vi "D2SParser - Private - Function - Open File.vi"(8 "error in (no error)":errorcluster, 10 "Path":path, 11 "D2SParser in":refnum<class "D2SParser.lvclass">) -> (0 "error out":errorcluster, 3 "D2SParser out":refnum<class "D2SParser.lvclass">)   [LabVIEW 2015, in "D2SParser.lvclass"]
uses:
  D2SParser.lvclass
  D2SParser.lvclass/D2SParser.ctl
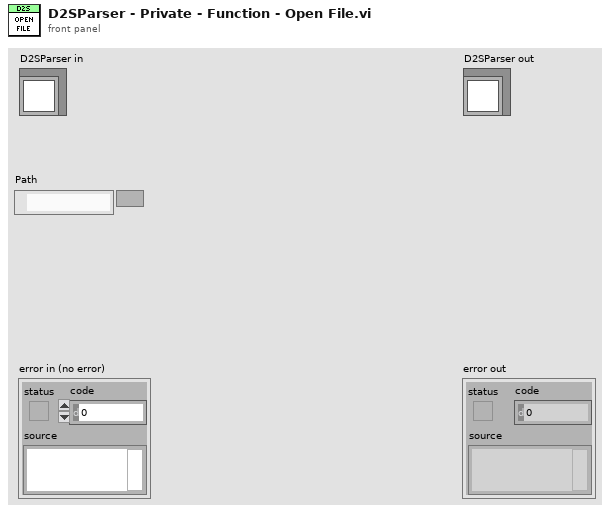
[diagram p1: front panel]
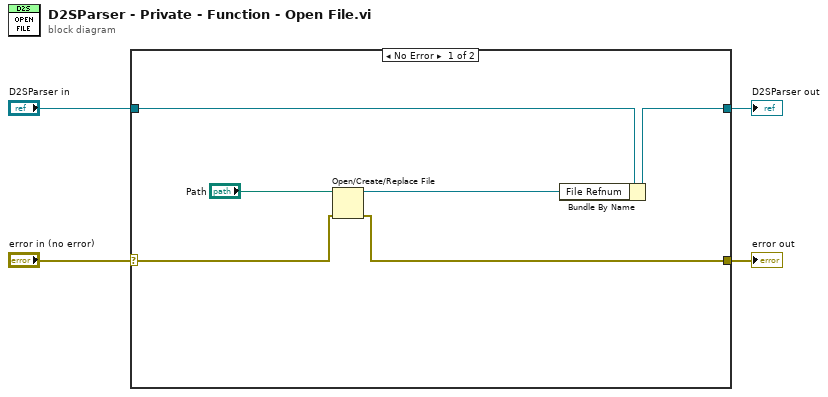
[diagram p0: block diagram]
diagram:
  n1 = case shown="No Error" "error in (no error)" {
    selector: "error in (no error)" -> [w8 w12]
    tunnel: [w7 w12] -> w3
    tunnel: [w6 w11] -> w1
    tunnel: "D2SParser in" -> [w10 w11]
    frame No Error {
      n2 = Open/Create/Replace File(file path (use dialog)="Path", error in=w8) -> (refnum out=w5:refnum<file>, error out=w7:errorcluster)  [unwired: 4 in, 1 out]
      n3 = Bundle By Name(cluster=w10, "File Refnum"=w5) -> (w6:refnum<class "D2SParser.lvclass">)
    }
    frame Error {
    }
  }
  "error out" <- w3
  "D2SParser out" <- w1
